vi "emi_Is App Closing.vi"(9 "error in (no error)":errorcluster) -> (10 "error out":errorcluster, 13 "App Close?":bool)   [LabVIEW 2011]
doc: "Checks wheter the application id closeing,"
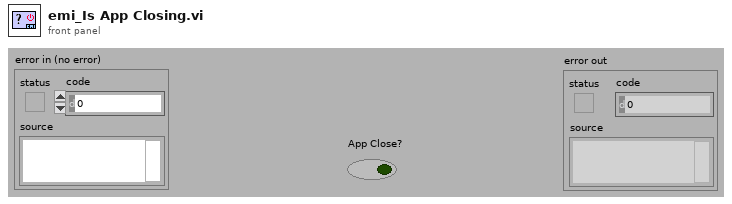
[diagram p1: front panel]
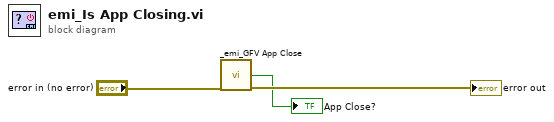
[diagram p0: block diagram]
diagram:
  n1 = call "_emi_GFV App Close.vi"("error in (no error)"="error in (no error)") -> ("App Close out"=→"App Close?":bool, "error out"=→"error out":errorcluster)  [unwired: 13 in]
